vi "DSF.Shared.Configuration.Cycle Timed.Set Priority.vi"(8 "error in (no error)":errorcluster, 10 "Priority":u8, 11 "Cycle Timed Configuration in":refnum<class "DSF.Shared.Configuration.Cycle Timed.lvclass">) -> (0 "error out":errorcluster, 3 "Cycle Timed Configuration out":refnum<class "DSF.Shared.Configuration.Cycle Timed.lvclass">)   [LabVIEW 2016, in "DSF.Shared.lvlib" / "DSF.Shared.Configuration.Cycle Timed.lvclass"]
uses:
  DSF.Shared.Configuration.Cycle Timed.lvclass
  DSF.Shared.Configuration.Cycle Timed.lvclass/DSF.Shared.Configuration.Cycle Timed.ctl
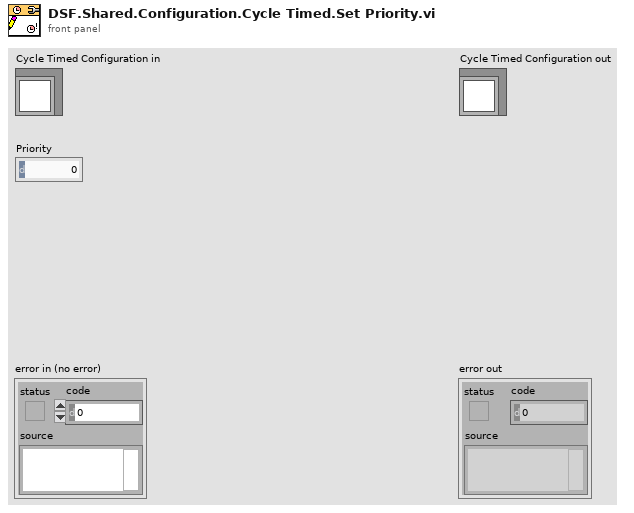
[diagram p1: front panel]
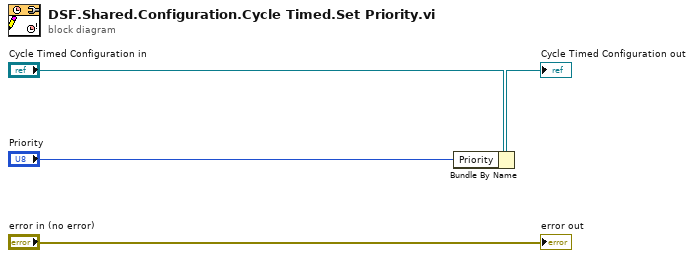
[diagram p0: block diagram]
diagram:
  n1 = Bundle By Name(cluster="Cycle Timed Configuration in", "Priority"="Priority") -> (→"Cycle Timed Configuration out":refnum<class "DSF.Shared.Configuration.Cycle Timed.lvclass">)
  "error out" <- "error in (no error)"
